vi "timestring.vi"(8 "error in (no error)":errorcluster, 10 "String Array In":string[](array[string])) -> (0 "error out":errorcluster, 2 "Time Stamp Out":timestamp[](array[timestamp]) format="%<%X>T")   [LabVIEW 2017]
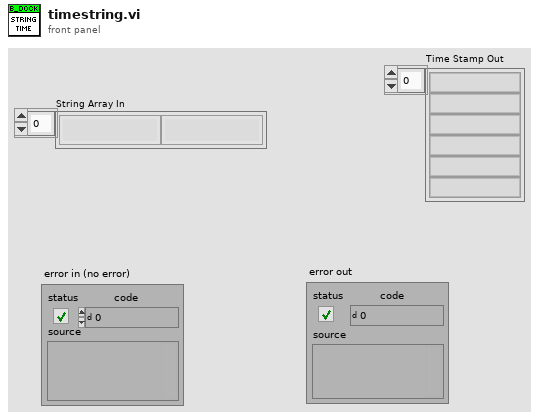
[diagram p1: front panel]
types:
  T1 = cluster{"second":i32, "minute":i32, "hour":i32, "day of month":i32, "month":i32, "year":i32, "day of week":i32, "day of year":i32, "is DST":i32}
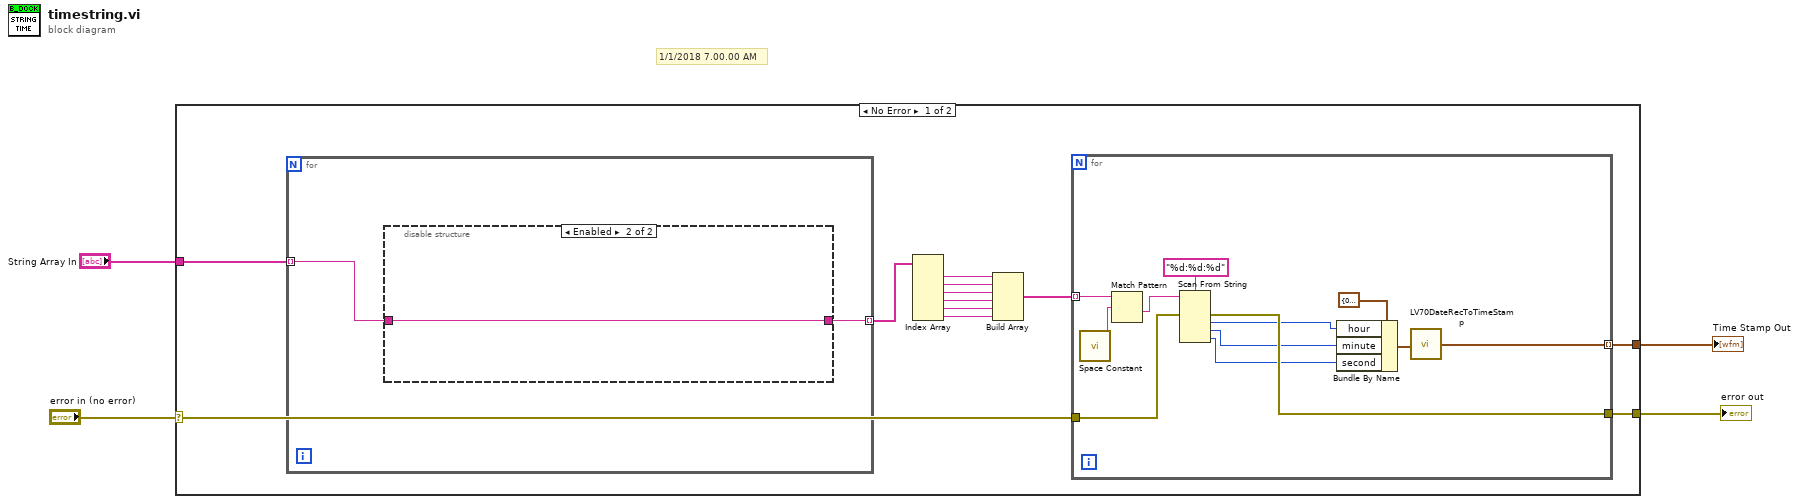
[diagram p0: block diagram]
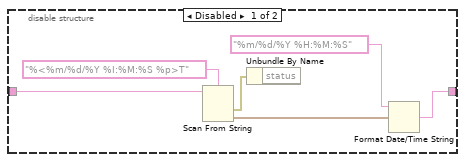
[diagram p2: hidden frame]
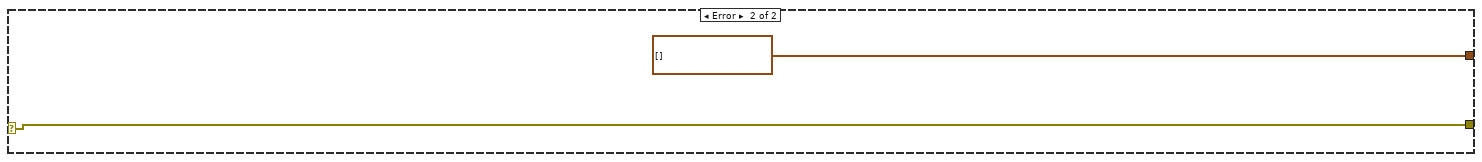
[diagram p3: hidden frame]
diagram:
  # "1/1/2018 7.00.00 AM"
  n1 = case shown="No Error" "error in (no error)" {
    selector: "error in (no error)" -> [w10 w39]
    tunnel: "String Array In" -> [w6 _]
    tunnel: [w12 timestamp[] []] -> w3
    tunnel: [w9 w39] -> w1
    frame No Error {
      n2 = for {
        tunnel: w6 -> [w17] mode=indexing
        tunnel: [w18] -> w5 mode=indexing
        n3 = disable-structure shown="Enabled" {
          disable-tunnel: [w20 w25] -> w18
          disable-tunnel: w17 -> [w19 w25]
          frame Disabled {
            n4 = Scan From String(format string="%<%m/%d/%Y %I:%M:%S %p>T", input string=w19) -> (error out=w21:errorcluster, output 1=w23:timestamp)  [unwired: 3 in, 2 out]
            n5 = Unbundle By Name(w21) -> ()  [unwired: 1 out]
            n6 = Format Date/Time String(time format string (%c)="%m/%d/%Y %H:%M:%S", seconds (now)=w23) -> (date/time string=w20:string)  [unwired: 1 in]
          }
          frame Enabled {
          }
        }
      }
      n7 = Index Array(array=w5) -> (element #1=w7:string, element #2=w16:string, element #3=w15:string, element #4=w14:string, element #5=w13:string, element #6=w11:string)  [unwired: 6 in]
      n8 = Build Array(w7, w16, w15, w14, w13, w11) -> (w8:string[])
      n9 = for {
        tunnel: w8 -> [w32] mode=indexing
        tunnel: [w36] -> w12 mode=indexing
        tunnel: w10 -> [w35]
        tunnel: [w34] -> w9
        n10 = call <vilib>:"Space Constant.vi"() -> ("String"=w33:string)
        n11 = Match Pattern(string=w32, regular expression=w33) -> (after substring=w31:string)  [unwired: 1 in, 3 out]
        n12 = Scan From String(format string="%d:%d:%d", input string=w31, error in=w35) -> (error out=w34:errorcluster, output 1=w28:i32, output 2=w27:i32, output 3=w26:i32)  [unwired: 4 in, 2 out]
        n13 = Bundle By Name(cluster=T1 {"second"=0, "minute"=0, "hour"=0, "day of month"=1, "month"=1, "year"=2018, "day of week"=0, "day of year"=0, "is DST"=0} ("date time rec"), "hour"=w28, "minute"=w27, "second"=w26) -> (w30:T1)
        n14 = call <vilib>:"LV70DateRecToTimeStamp.vi"("date time rec"=w30) -> ("Time Stamp"=w36:timestamp)
      }
    }
    frame Error {
    }
  }
  "Time Stamp Out" <- w3
  "error out" <- w1
